vi "RQST Comm Lookup Table_Initialize.vi"(8 "error in (no error)":errorcluster) -> (0 "error out":errorcluster {"code" min=0 max=0}, 3 "vi reference":T1)   [LabVIEW 2015, in "Diagnostics Addon Engine.lvlib"]
uses:
  Diagnostics Addon Engine.lvlib
  STM Lookup Table Ref.ctl
  Connection Manager/stm_TCPConnectionMethod.ctl
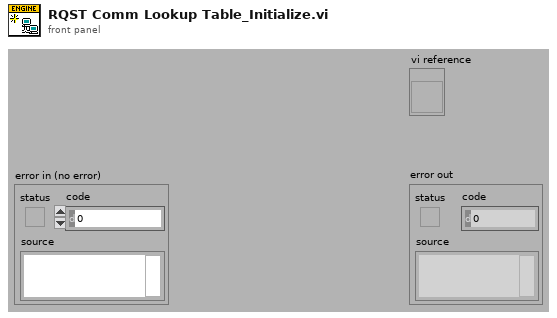
[diagram p1: front panel]
types:
  T1 = typedef "Diagnostics Addon Engine.lvlib/STM Lookup Table Ref.ctl" = refnum<vi>
  T2 = typedef "Diagnostics Addon Engine.lvlib/stm_TCPConnectionMethod.ctl" = enum16{"Initialize", "Add Connection", "Set Properties", "Get Connection(s)", "Remove Connection", "Remove All Connections", "Get Connection Count"}
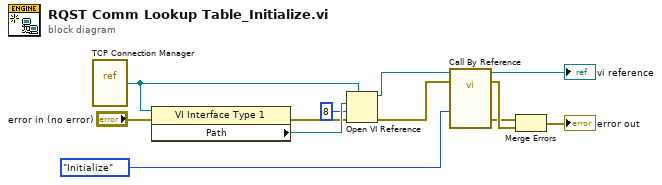
[diagram p0: block diagram]
diagram:
  n1 = vi-ref "TCP Connection Manager.vi"() -> (w7:refnum<vi>)
  n2 = property class="VI Interface Type 1"(reference=w7, error in="error in (no error)") -> (error out=w10:errorcluster, "Path"=w12:path)  [unwired: 1 out]
  n3 = Open VI Reference(type specifier VI Refnum (for type only)=w7, vi path=w12, options=8, error in (no error)=w10) -> (vi reference=w6:refnum<vi>, error out=w5:errorcluster)  [unwired: 2 in]
  n4 = call-by-ref "?"(reference=w6, error in=w5, "Method"=stm_TCPConnectionMethod."Initialize") -> (reference out=→"vi reference":refnum<vi>, error out=w3:errorcluster, 0:"error out"=w2:errorcluster)  [unwired: 5 in, 5 out]
  n5 = Merge Errors(w2, w3) -> (→"error out":errorcluster)
